vi "iviDMMtest.vi"() -> ()   [LabVIEW 2020]
panel:
  in  "logical name":refnum<k15>="Multimeter" caption="logical name (\"SampleDmm\")"
  out "error out":errorcluster {"code" format="%.0x"}
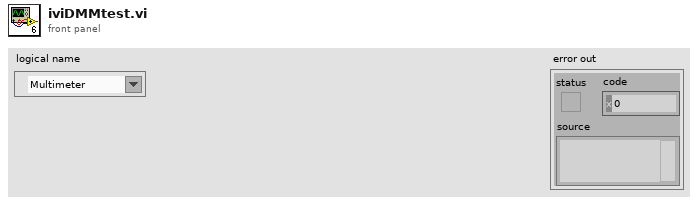
[diagram p1: front panel]
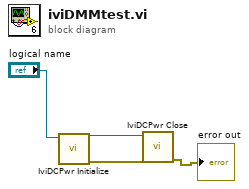
[diagram p0: block diagram]
diagram:
  n1 = call <vilib>:"IviDCPwr Initialize.vi"("logical name (\"SamplePowerSupply\")"="logical name") -> ("error out"=w3:errorcluster, "instrument handle"=w4:refnum<k15>)  [unwired: 9 in]
  n2 = call <vilib>:"IviDCPwr Close.vi"("error in (no error)"=w3, "instrument handle"=w4) -> ("error out"=→"error out":errorcluster)  [unwired: 9 in]
